vi "place sensor on baseplate.vi"() -> ()   [LabVIEW 2018]
uses:
  Classes/Workspace/Component/Component Tray.lvclass
  Classes/Controller/Controller.lvclass
  Classes/Routine/Pick and Place/Pick and Place.lvclass
  Classes/Routine/Pick and Place/Pick and Place Type.ctl
  Classes/Workspace/Pick Up Tool Area/Pick Up Tool Fixture.lvclass
  Classes/Workspace/Carrier Tray/Assembly Tray.lvclass
panel:
  out "error out":errorcluster
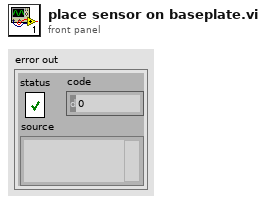
[diagram p1: front panel]
types:
  T1 = typedef "Pick and Place.lvclass/Pick and Place Type.ctl" = enum16{"Primary Pick Up", "Secondary Pick Up", "Put Down All", "Pick Up All", "Put Down Secondary"}
  T2 = typedef "Controller.lvclass/Controllers.ctl" = cluster{"I-O.lvclass":refnum<class "I-O.lvclass">, "Gantry":refnum<k24>, "Dispenser":refnum<visa-resource-name>}
  T3 = typedef "Fixture.lvclass/Workspace.ctl" = cluster{"XYZTheta":dbl[], "Workspace Valve":i32, "Workspace Sensor":i32}
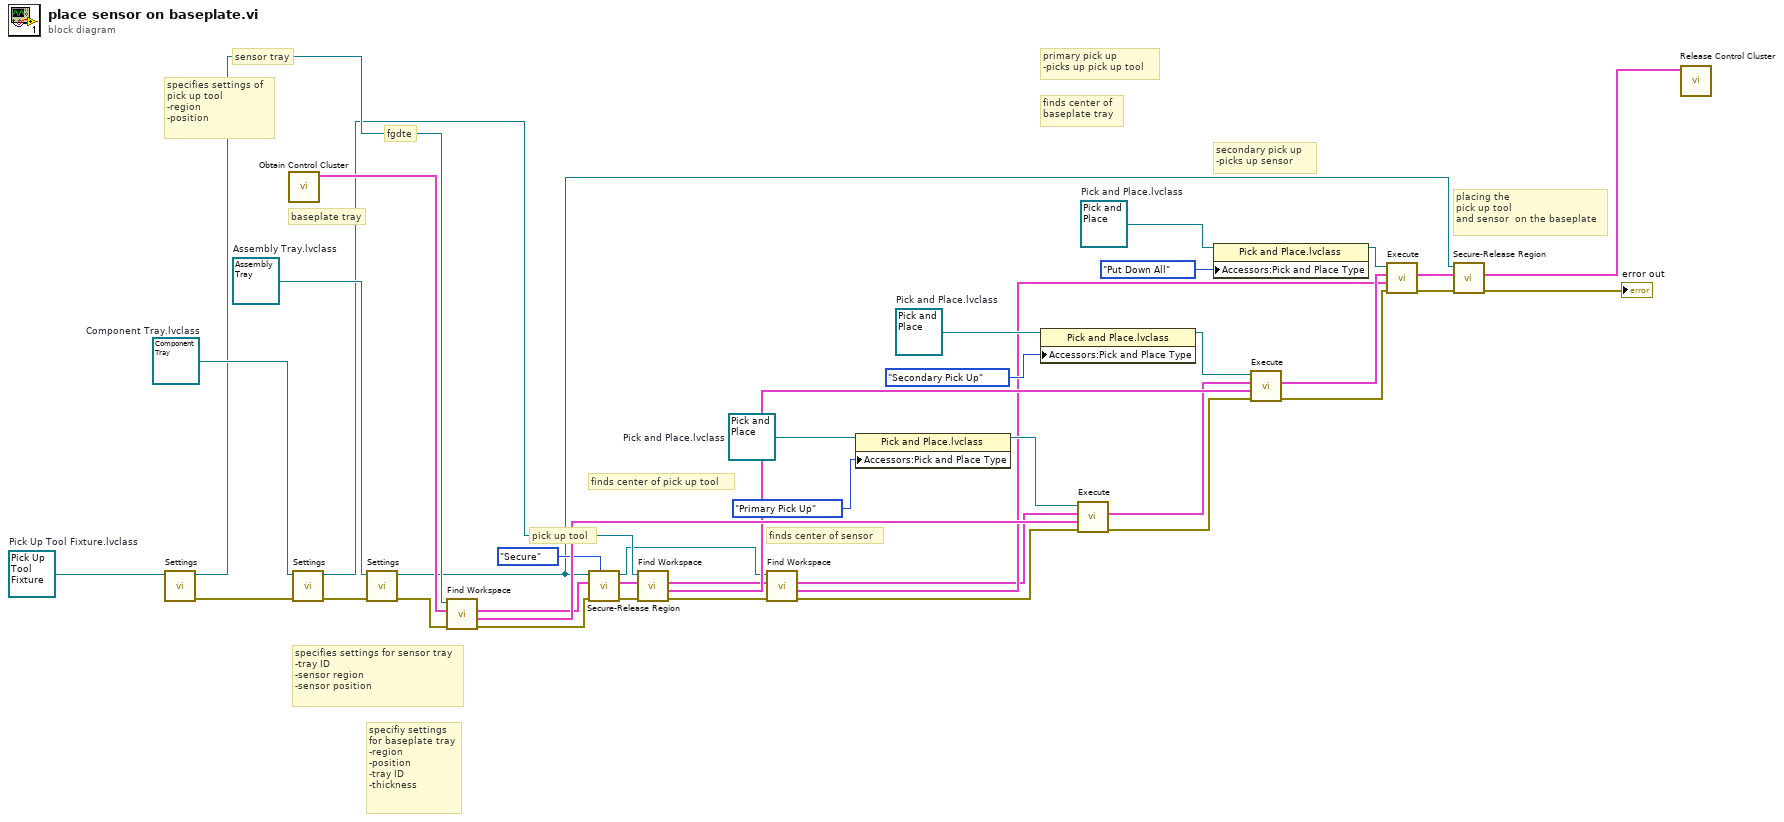
[diagram p0: block diagram]
diagram:
  w22 = refnum<class "Pick and Place.lvclass"> refnum  # Pick and Place.lvclass
  w24 = refnum<class "Assembly Tray.lvclass"> refnum  # Assembly Tray.lvclass
  w33 = refnum<class "Pick and Place.lvclass"> refnum  # Pick and Place.lvclass
  w36 = refnum<class "Pick Up Tool Fixture.lvclass"> refnum  # Pick Up Tool Fixture.lvclass
  w39 = refnum<class "Pick and Place.lvclass"> refnum  # Pick and Place.lvclass
  w40 = refnum<class "Component Tray.lvclass"> refnum  # Component Tray.lvclass
  # "fgdte"
  # "finds center of \nbaseplate tray"
  # "specifiy settings \nfor baseplate tray\n-region\n-position\n-tray ID\n-thickness"
  # "placing the \npick up tool \nand sensor  on the baseplate"
  # "baseplate tray"
  # "secondary pick up \n-picks up sensor"
  # "primary pick up\n-picks up pick up tool"
  # "finds center of sensor"
  # "finds center of pick up tool"
  # "specifies settings for sensor tray\n-tray ID\n-sensor region\n-sensor position"
  # "specifies settings of \npick up tool\n-region\n-position"
  # "pick up tool"
  # "sensor tray"
  n1 = call-dynamic "Settings.vi"("Workspace in"=w36) -> ("error out"=w30:errorcluster, "Workspace out"=w35:refnum<class "Pick Up Tool Fixture.lvclass">)  [unwired: 9 in]
  n2 = call "Obtain Control Cluster.vi"() -> ("Control Out"=w34:T2)  [unwired: 11 in]
  n3 = call-dynamic "Settings.vi"("error in (no error)"=w30, "Component in"=w40) -> ("error out"=w26:errorcluster, "Component out"=w16:refnum<class "Component Tray.lvclass">)  [unwired: 8 in]
  n4 = call-dynamic "Settings.vi"("error in (no error)"=w26, "Assembly Tray In"=w24) -> ("error out"=w25:errorcluster, "Assembly Tray Out"=w3:refnum<class "Assembly Tray.lvclass">)  [unwired: 8 in]
  n5 = call-dynamic "Find Workspace.vi"("Error In"=w25, "Control In"=w34, "Workspace In"=w35) -> ("Error Out"=w8:errorcluster, "Workspace Out"=w29:T3, "Control Out"=w10:T2)  [unwired: 5 in, 1 out]
  n6 = call-dynamic "Secure-Release Region.vi"("Action"=enum16{"Secure", "Release"}."Secure", "error in (no error)"=w8, "Control In"=w10, "Carrier Tray in"=w3) -> ("error out"=w7:errorcluster, "Control Out"=w9:T2, "Carrier Tray out"=w11:refnum<class "Assembly Tray.lvclass">)  [unwired: 5 in]
  n7 = call-dynamic "Find Workspace.vi"("error in (no error)"=w7, "Control In"=w9, "Component.lvclass"=w16) -> ("error out"=w15:errorcluster, "Workspace"=w28:T3, "Control Out"=w23:T2)  [unwired: 5 in, 1 out]
  n8 = call-dynamic "Find Workspace.vi"("Error In"=w15, "Control In"=w23, "Carrier Tray in"=w11) -> ("Error Out"=w14:errorcluster, "Workspace"=w18:T3, "Control Out"=w17:T2)  [unwired: 5 in, 1 out]
  n9 = property class="Pick and Place.lvclass"(reference=w33, "Accessors:Pick and Place Type"=Pick_and_Place_Type."Primary Pick Up" ("Pick and Place Type")) -> (reference out=w31:refnum<class "Pick and Place.lvclass">)  [unwired: 1 in, 1 out]
  n10 = property class="Pick and Place.lvclass"(reference=w39, "Accessors:Pick and Place Type"=Pick_and_Place_Type."Secondary Pick Up" ("Pick and Place Type")) -> (reference out=w37:refnum<class "Pick and Place.lvclass">)  [unwired: 1 in, 1 out]
  n11 = call-dynamic "Execute.vi"("error in (no error)"=w14, "Workspace"=w29, "Cluster"=w17, "Pick and Place in"=w31) -> ("error out"=w13:errorcluster, "Control Out"=w27:T2)  [unwired: 5 in, 1 out]
  n12 = property class="Pick and Place.lvclass"(reference=w22, "Accessors:Pick and Place Type"=Pick_and_Place_Type."Put Down All" ("Pick and Place Type")) -> (reference out=w21:refnum<class "Pick and Place.lvclass">)  [unwired: 1 in, 1 out]
  n13 = call-dynamic "Execute.vi"("error in (no error)"=w13, "Workspace"=w28, "Cluster"=w27, "Pick and Place in"=w37) -> ("error out"=w12:errorcluster, "Control Out"=w19:T2)  [unwired: 5 in, 1 out]
  n14 = call-dynamic "Execute.vi"("error in (no error)"=w12, "Workspace"=w18, "Cluster"=w19, "Pick and Place in"=w21) -> ("error out"=w2:errorcluster, "Control Out"=w5:T2)  [unwired: 5 in, 1 out]
  n15 = call-dynamic "Secure-Release Region.vi"("error in (no error)"=w2, "Control In"=w5, "Carrier Tray in"=w3) -> ("error out"=→"error out":errorcluster, "Control Out"=w4:T2)  [unwired: 6 in, 1 out]
  n16 = call "Release Control Cluster.vi"("output cluster"=w4) -> ()  [unwired: 11 in]
